vi "Package.vi"   [LabVIEW 2017, in "Scripts.lvlib"]
uses:
  Scripts.lvlib
  <vilib>/Field R&D Services/Labricator/Controls/LabVIEW Versions.ctl
  <vilib>/Field R&D Services/Labricator/Labricator.lvlib
types:
  T1 = typedef "Labricator.lvlib/LabVIEW Versions.ctl" = enum16{"2014", "2015", "2016", "2017", "2018"}
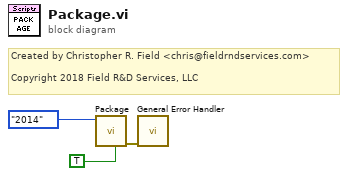
[diagram p0: block diagram]
diagram:
  # "Created by Christopher R. Field <chris@fieldrndservices.com>\n\nCopyright 2018 Field R&D Services, LLC"
  n1 = call <vilib>:"Package.vi"("Pre-Clean"=TRUE, "LabVIEW Previous Version"=LabVIEW_Versions."2014") -> ("Error Out"=w1:errorcluster)  [unwired: 9 in]
  n2 = call <vilib>:"General Error Handler.vi"("error in (no error)"=w1) -> ()  [unwired: 10 in, 5 out]
